vi "Get PWMout references.vi"(8 "error in (no error)":errorcluster, 10 "PWM out data":T2[](array[typedef]), 11 "Refnum in":refnum<k20>) -> (0 "error out":errorcluster, 2 "PWM out data":T1[](array[typedef]), 3 "Refnum out":refnum<k20>)   [LabVIEW 2013, in "PWM Engine.lvlib"]
uses:
  PWM Engine.lvlib
  Shared/Types/PWM out info.ctl
  Shared/Types/PWM out info(RT).ctl
  <vilib>/NI/LVFPGA Adv Session Resources/OpenByNameSubVI.vi
  <vilib>/rvi/interface/common/dynamic/niFpgaEscapeDelimiterAndNull.vi
  <vilib>/Utility/error.llb/Error Cluster From Error Code.vi
  <vilib>/NI/LVFPGA Adv Session Resources/OpenByName.xnode
  Shared/PWM Shared.lvlib
  <vilib>/NI/LVFPGA Adv Session Resources/LVFPGAAdvSessionResources.lvlib
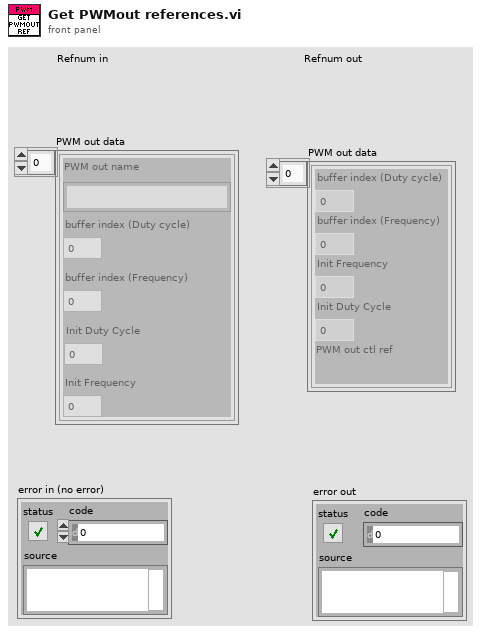
[diagram p1: front panel]
types:
  T1 = typedef "PWM Shared.lvlib/PWM out info(RT).ctl" = cluster{"buffer index (Duty cycle)":i32, "buffer index (Frequency)":i32, "Init Frequency":dbl, "Init Duty Cycle":dbl, "PWM out ctl ref":refnum<k20>}
  T2 = typedef "PWM Shared.lvlib/PWM out info.ctl" = cluster{"PWM out name":string, "buffer index (Duty cycle)":i32, "buffer index (Frequency)":i32, "Init Frequency":dbl, "Init Duty Cycle":dbl}
  T3 = cluster{"Name":string, "Depth":u32, "Write? (Deprecated:Use Implementation)":bool, "Physical Channel":u32, "Base Address":u32, "Data Width":u32, "Data Type":enum32{"Boolean", "I8", "I16", "I32", "I64", "U8", "U16", "U32", "U64", "FXP", "CustomControl", "SGL"}, "FXP Properties":variant, "Write Window Address":u32, "Implementation":enum16{"niFpgaTargetToHost", "niFpgaHostToTarget", "niFpgaPeerToPeerWriter", "niFpgaPeerToPeerReader", "niCoreTargetToHost", "niCoreHostToTarget"}, "Control Set":u32}[]
  T4 = cluster{"Name":string, "type":variant, "indicator?":bool}[]
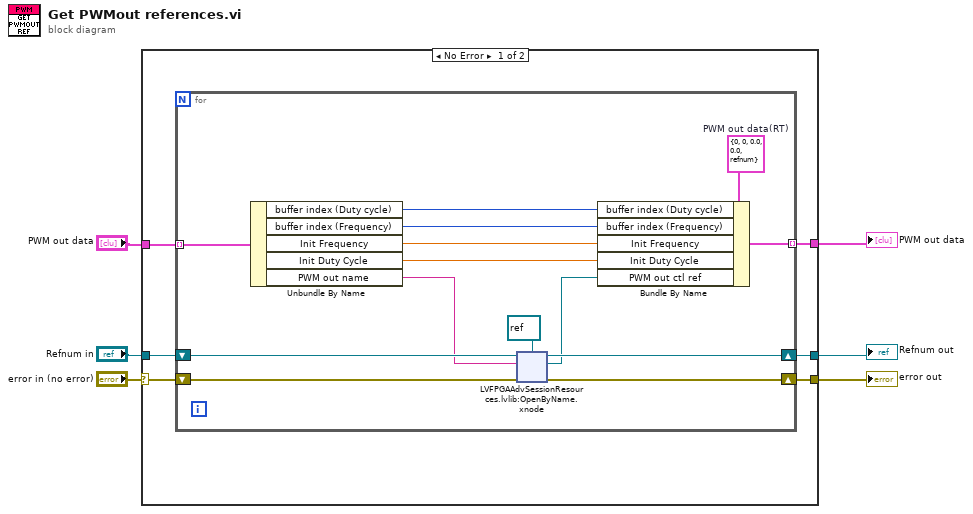
[diagram p0: block diagram]
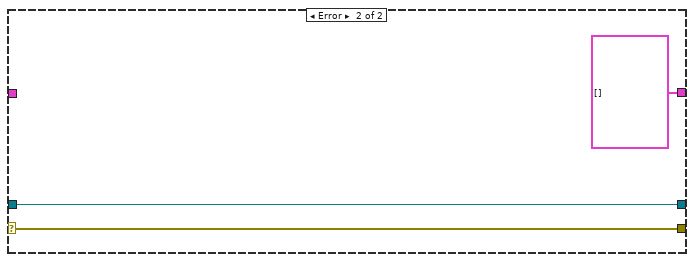
[diagram p2: hidden frame]
diagram:
  n1 = case shown="No Error" "error in (no error)" {
    selector: "error in (no error)" -> [w7 w42]
    tunnel: "Refnum in" -> [w12 w41]
    tunnel: [w11 w42] -> w5
    tunnel: [w10 T1[] []] -> w4
    tunnel: [w9 w41] -> w3
    tunnel: "PWM out data" -> [w8 _]
    frame No Error {
      n2 = for {
        shift-right: [w23] -> w9
        shift-left: w12 -> [w26]
        shift-right: [w24] -> w11
        shift-left: w7 -> [w25]
        tunnel: w8 -> [w22] mode=indexing
        tunnel: [w21] -> w10 mode=indexing
        w19 = T1 {"buffer index (Duty cycle)"=0, "buffer index (Frequency)"=0, "Init Frequency"=0.0, "Init Duty Cycle"=0.0, "PWM out ctl ref"=refnum}  # PWM out data(RT)
        n3 = Unbundle By Name(w22) -> ("buffer index (Duty cycle)"=w17:i32, "buffer index (Frequency)"=w16:i32, "Init Frequency"=w15:dbl, "Init Duty Cycle"=w14:dbl, "PWM out name"=w20:string)
        n4 = xnode "LVFPGAAdvSessionResources.lvlib:OpenByName.xnode"("FPGA VI Reference in"=w26, "Resource name in"=w20, "Single resource reference type in"=refnum<k20> refnum ("FPGA Interface"), "Error in"=w25) -> ("Single resource reference out"=w18:refnum<k20>, "Error out"=w24:errorcluster, "FPGA VI Reference out"=w23:refnum<k20>)
        n5 = Bundle By Name(cluster=w19, "buffer index (Duty cycle)"=w17, "buffer index (Frequency)"=w16, "Init Frequency"=w15, "Init Duty Cycle"=w14, "PWM out ctl ref"=w18) -> (w21:T1)
      }
    }
    frame Error {
    }
  }
  "PWM out data" <- w4
  "Refnum out" <- w3
  "error out" <- w5
